vi "command_processor.vi"(8 "error in (no error)":errorcluster) -> (0 "error out":errorcluster)   [LabVIEW 2021]
uses:
  FGVs/FGVstates.ctl
  <vilib>/sound2/lvsound2.llb/Sampling Mode.ctl
  FGVs/AppStates.ctl
  <vilib>/sound2/lvsound2.llb/Sound Output Task ID.ctl
  <vilib>/sound2/lvsound2.llb/Sound File Position.ctl
  <vilib>/sound2/lvsound2.llb/Sound File Info (path).vi
  <vilib>/sound2/lvsound2.llb/Sound File Read Open.vi
  <vilib>/sound2/lvsound2.llb/Sound File Read (DBL).vi
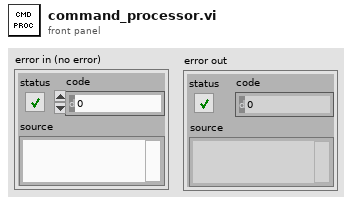
[diagram p1: front panel]
types:
  T1 = typedef "FGVstates.ctl" = enum16{"Init", "Set", "Get", "De-Init"}
  T2 = typedef "settings.ctl" = cluster{"scan_dir_path":path, "Number of Samples/Iteration":i32}
  T3 = typedef "data_exchange_fgv.ctl" = cluster{"queue states":refnum<queue>, "audio data":refnum<queue>, "error queue":refnum<queue>}
  T4 = typedef "AppStates.ctl" = enum16{"Init", "Scan Music Dir", "Idle", "Playback", "Enqueue samples", "Pause playback", "Stop playback", "Exit"}
  T5 = typedef "Sound Output Task ID.ctl" = u32
  T6 = typedef "ButtonRefs.ctl" = cluster{"Button_play":refnum<vi>, "Button_pause":refnum<vi>, "Button_stop":refnum<vi>, "Playback status":refnum<vi>, "Playback Timeline":refnum<vi>, "Right Channel":refnum<vi>, "Left Channel":refnum<vi>, "Skip Forward Button":refnum<vi>, "Skip Back Button":refnum<vi>, "Playlist":refnum<vi>}
  T7 = typedef "Sampling Mode.ctl" = i32
  T8 = typedef "Sound Data Format.ctl" = cluster{"sample rate (S/s)":dbl, "number of channels":i32, "bits per sample":i32}
  T9 = typedef "Sound File Refnum.ctl" = refnum<file>
  T10 = typedef "Sound File Position.ctl" = u16
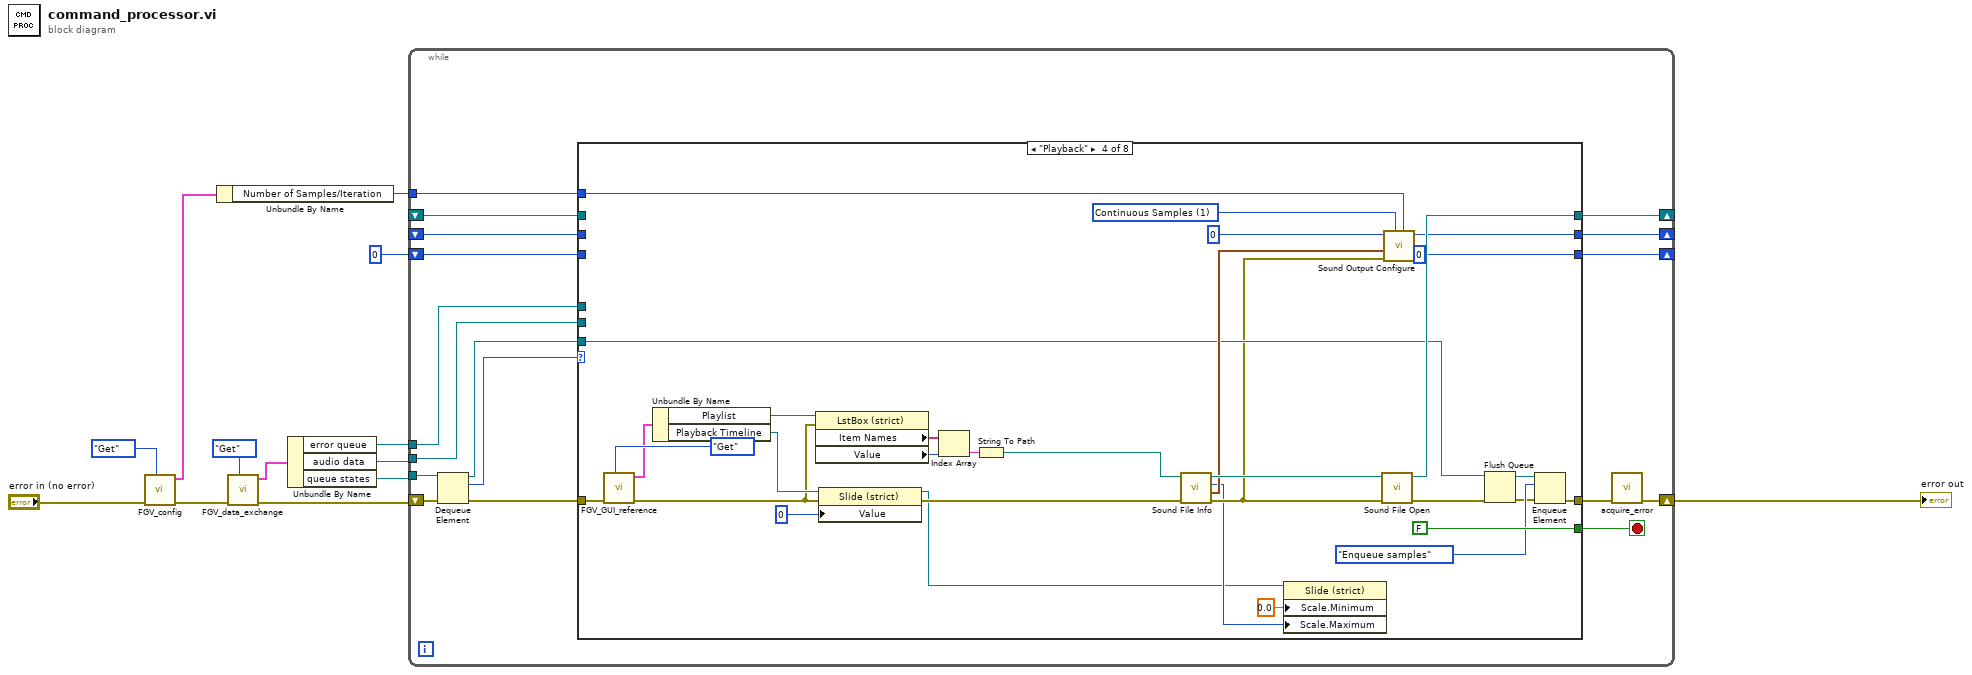
[diagram p0: block diagram]
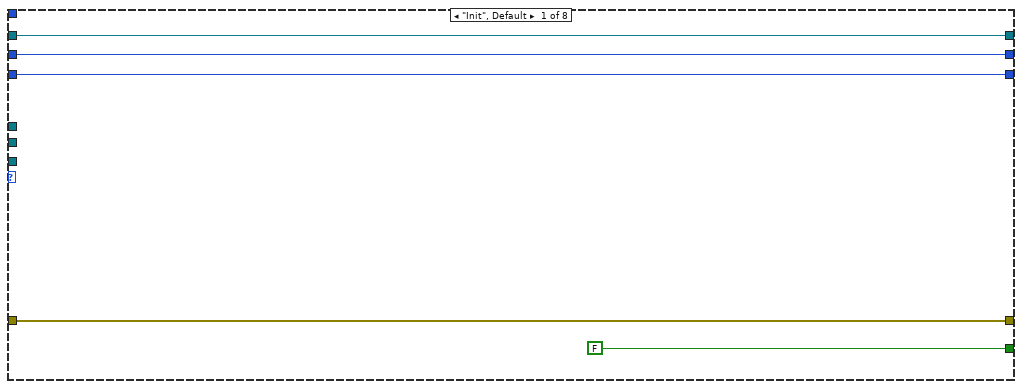
[diagram p2: hidden frame]
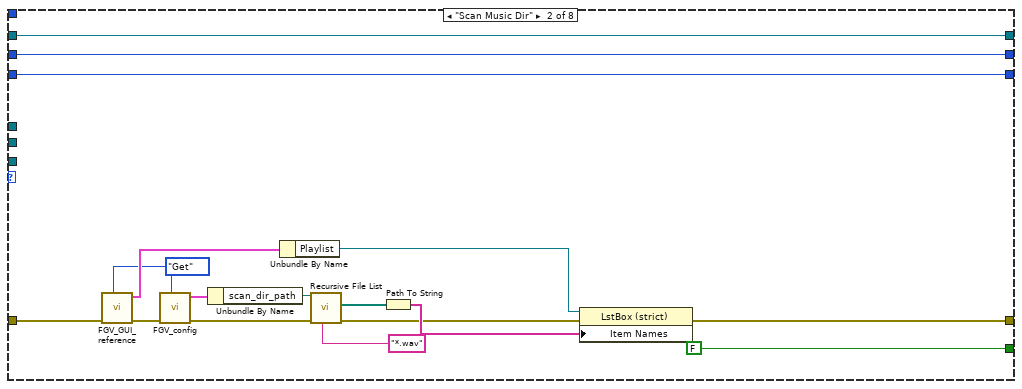
[diagram p3: hidden frame]
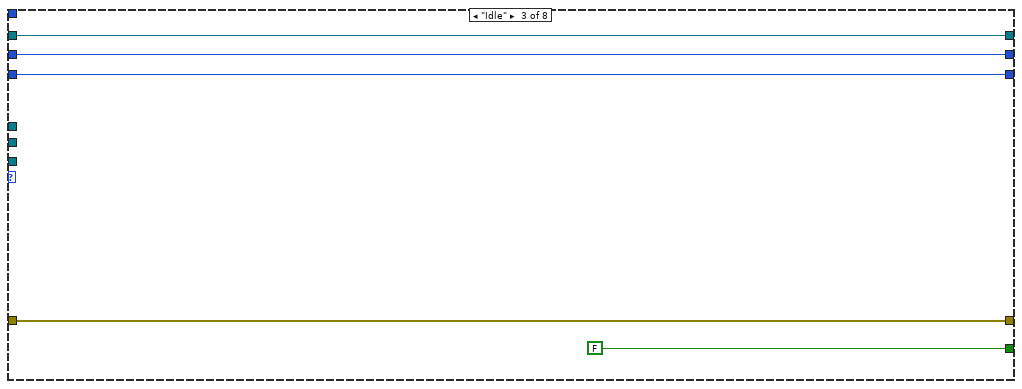
[diagram p4: hidden frame]
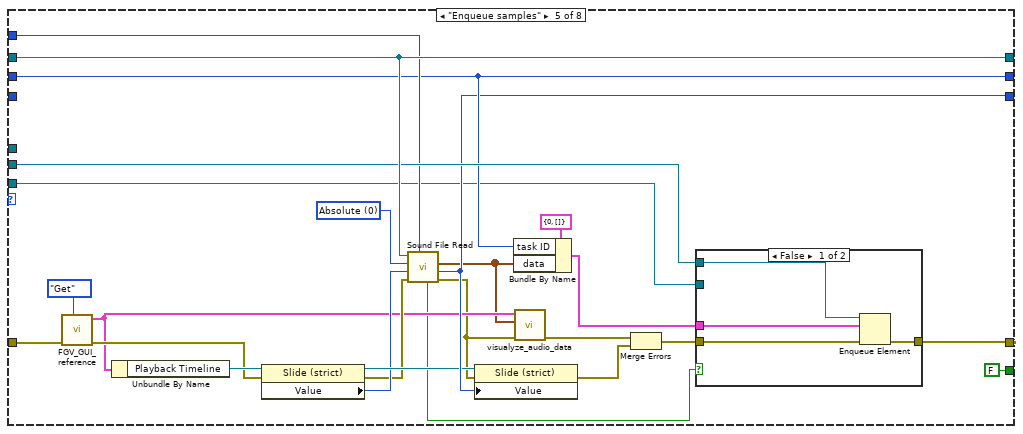
[diagram p5: hidden frame]
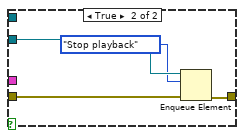
[diagram p6: hidden frame]
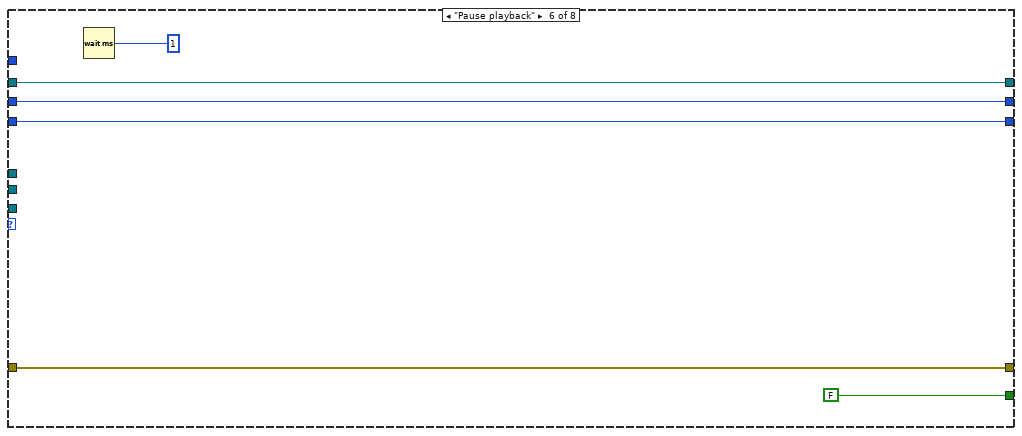
[diagram p7: hidden frame]
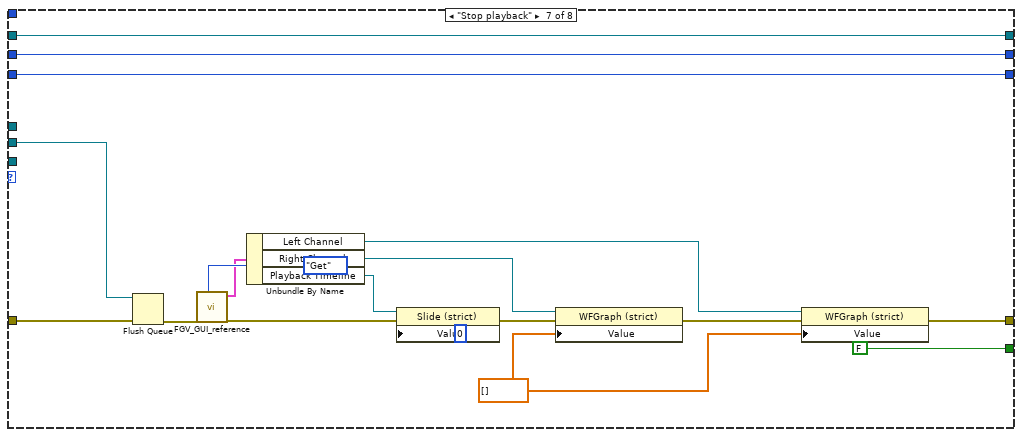
[diagram p8: hidden frame]
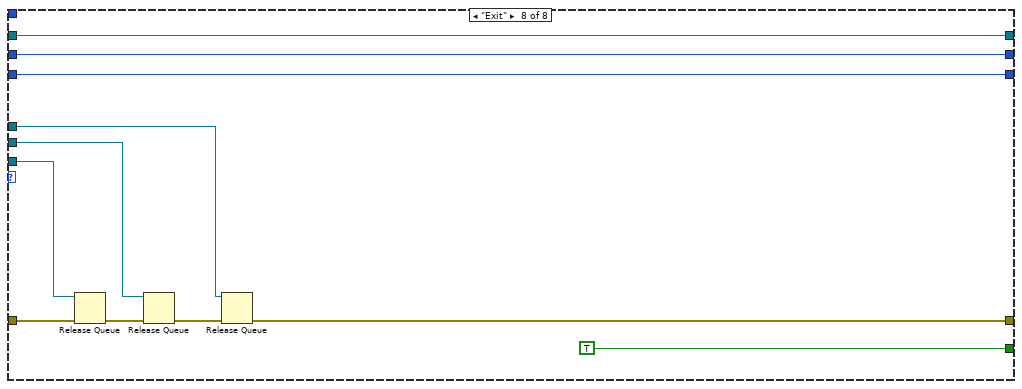
[diagram p9: hidden frame]
diagram:
  n1 = call "FGV_config.vi"("FGV states"=FGVstates."Get", "error in (no error)"="error in (no error)") -> ("error out"=w4:errorcluster, "Settings"=w2:T2)  [unwired: 8 in]
  n2 = Unbundle By Name(w2) -> ("Number of Samples/Iteration"=w1:i32)
  n3 = call "FGV_data_exchange.vi"("FGV states"=FGVstates."Get", "error in (no error)"=w4) -> ("error out"=w10:errorcluster, "main_cycle_queue"=w11:T3)  [unwired: 8 in]
  n4 = Unbundle By Name(w11) -> ("error queue"=w6:refnum<queue>, "audio data"=w8:refnum<queue>, "queue states"=w9:refnum<queue>)
  n5 = while {
    shift-right: [w15] -> w13
    shift-left: w10 -> [w30]
    tunnel: w9 -> [w26]
    shift-right: [w25] -> _
    shift-left: _ -> [w24]
    shift-right: [w23] -> _
    shift-left: _ -> [w22]
    tunnel: w1 -> [w20]
    tunnel: w8 -> [w19]
    shift-right: [w17] -> _
    shift-left: 0 ("position offset") -> [w18]
    tunnel: w6 -> [w14]
    stop <- w27 stop-if-true
    n6 = Dequeue Element(queue=w26, error in (no error)=w30) -> (queue out=w21:refnum<queue>, element=w29:T4, error out=w28:errorcluster)  [unwired: 1 in, 1 out]
    n7 = case shown="\"Playback\"" w29 {
      tunnel: w28 -> [w35 w50 w57 w88 w103 w122 w129 w152]
      tunnel: [w35 w36 w57 w74 w106 w122 w133 w146] -> w16
      tunnel: [FALSE FALSE FALSE FALSE FALSE FALSE FALSE TRUE] -> w27
      tunnel: [w32 w44 w54 w78 w112 w127 w145 w155] -> w25
      tunnel: w24 -> [w32 w44 w54 _ w112 w127 w145 w155]
      tunnel: [w33 w45 w55 w75 w108 w126 w144 w154] -> w23
      tunnel: w22 -> [w33 w45 w55 _ w108 w126 w144 w154]
      tunnel: w21 -> [_ _ _ w65 w89 _ _ w150]
      tunnel: w20 -> [_ _ _ w72 w110 _ _ _]
      tunnel: w19 -> [_ _ _ _ w111 _ w128 w149]
      tunnel: w18 -> [w31 w43 w53 _ _ w123 w143 w153]
      tunnel: [w31 w43 w53 0 ("position offset") w102 w123 w143 w153] -> w17
      tunnel: w14 -> [_ _ _ _ _ _ _ w147]
      frame "Init", Default {
      }
      frame "Scan Music Dir" {
        w41 = FGVstates."Get" ("FGV states")
        n8 = call "FGV_GUI_reference.vi"("FGV states"=w41, "error in (no error)"=w50) -> ("error out"=w42:errorcluster, "Button refs Out"=w49:T6)  [unwired: 8 in]
        n9 = call "FGV_config.vi"("FGV states"=w41, "error in (no error)"=w42) -> ("error out"=w40:errorcluster, "Settings"=w39:T2)  [unwired: 8 in]
        n10 = Unbundle By Name(w39) -> ("scan_dir_path"=w38:path)
        n11 = Unbundle By Name(w49) -> ("Playlist"=w46:refnum<vi>)
        n12 = call <vilib>:"Recursive File List.vi"("pattern"="*.wav", "error in (no error)"=w40, "Folder Path"=w38) -> ("error out"=w37:errorcluster, "All Files in Dir"=w48:path[])  [unwired: 4 in, 3 out]
        n13 = Path To String(path=w48) -> (string=w47:string[])
        n14 = property class="LstBox (strict)"(reference=w46, error in=w37, "Item Names"=w47) -> (error out=w36:errorcluster)  [unwired: 1 out]
      }
      frame "Idle" {
      }
      frame "Playback" {
        w77 = T7 1 items=["Finite Samples", "Continuous Samples"] ("sample mode")
        n15 = call "FGV_GUI_reference.vi"("FGV states"=FGVstates."Get", "error in (no error)"=w88) -> ("error out"=w64:errorcluster, "Button refs Out"=w86:T6)  [unwired: 8 in]
        n16 = Unbundle By Name(w86) -> ("Playlist"=w85:refnum<vi>, "Playback Timeline"=w69:refnum<vi>)
        n17 = property class="LstBox (strict)"(reference=w85, error in=w64) -> ("Item Names"=w82:string[], "Value"=w83:i32)  [unwired: 2 out]
        n18 = property class="Slide (strict)"(reference=w69, error in=w64, "Value"=0) -> (reference out=w58:refnum<vi>, error out=w63:errorcluster)
        n19 = Index Array(array=w82, index=w83) -> (element=w81:string)
        n20 = String To Path(string=w81) -> (path=w79:path)
        n21 = call-poly <vilib>:"Sound File Info.vi"("error in (no error)"=w63, "path"=w79) -> ("error out"=w62:errorcluster, "sound format"=w71:T8, "total number of samples/ch"=w59:u32, "path out"=w80:path)  [unwired: 6 in]
        n22 = property class="Slide (strict)"(reference=w58, "Scale.Minimum"=0.0 ("Scale.Range:Minimum"), "Scale.Maximum"=w59) -> ()  [unwired: 1 in, 2 out]
        n23 = call-poly <vilib>:"Sound File Open.vi"("error in (no error)"=w62, "path"=w80) -> ("error out"=w61:errorcluster, "sound file refnum"=w78:T9)  [unwired: 8 in]
        n24 = call <vilib>:"Sound Output Configure.vi"("number of samples/ch"=w72, "sample mode"=w77, "error in (no error)"=w62, "sound format"=w71, "device ID"=u32 0) -> ("task ID"=w75:T5)  [unwired: 5 in, 1 out]
        n25 = Flush Queue(queue=w65, error in (no error)=w61) -> (queue out=w66:refnum<queue>, error out=w67:errorcluster)  [unwired: 1 out]
        n26 = Enqueue Element(queue=w66, element=AppStates."Enqueue samples", error in (no error)=w67) -> (error out=w74:errorcluster)  [unwired: 1 in, 2 out]
      }
      frame "Enqueue samples" {
        w105 = T10 0 items=["Absolute"=0, "Relative"=2] ("position mode")
        n27 = call "FGV_GUI_reference.vi"("FGV states"=FGVstates."Get", "error in (no error)"=w103) -> ("error out"=w97:errorcluster, "Button refs Out"=w96:T6)  [unwired: 8 in]
        n28 = Unbundle By Name(w96) -> ("Playback Timeline"=w100:refnum<vi>)
        n29 = property class="Slide (strict)"(reference=w100, error in=w97) -> (reference out=w101:refnum<vi>, error out=w98:errorcluster, "Value"=w99:i32)
        n30 = call-poly <vilib>:"Sound File Read.vi"("number of samples/ch (-1: all)"=w110, "error in (no error)"=w98, "position offset"=w99, "position mode"=w105, "sound file refnum"=w112) -> ("error out"=w91:errorcluster, "offset"=w102:i32, "data"=w95:waveform(dbl)[], "end of file?"=w90:bool)  [unwired: 2 in, 1 out]
        n31 = property class="Slide (strict)"(reference=w101, error in=w91, "Value"=w102) -> (error out=w94:errorcluster)  [unwired: 1 out]
        n32 = Bundle By Name(cluster=cluster{"task ID":T5, "data":waveform(dbl)[]} {"task ID"=0, "data"=[]} ("element"), "task ID"=w108, "data"=w95) -> (w107:cluster{"task ID":T5, "data":waveform(dbl)[]})
        n33 = call "visualyze_audio_data.vi"("error in (no error)"=w91, "audio data"=w95, "Button refs In"=w96) -> ("error out"=w93:errorcluster)  [unwired: 8 in]
        n34 = Merge Errors(w93, w94) -> (w92:errorcluster)
        n35 = case shown="False" w90 {
          tunnel: w111 -> [w117 _]
          tunnel: w107 -> [w116 _]
          tunnel: [w115 w120] -> w106
          tunnel: w92 -> [w114 w118]
          tunnel: w89 -> [_ w121]
          frame False {
            n36 = Enqueue Element(queue=w117, element=w116, error in (no error)=w114) -> (error out=w115:errorcluster)  [unwired: 1 in, 2 out]
          }
          frame True {
            n37 = Enqueue Element(queue=w121, element=AppStates."Stop playback", error in (no error)=w118) -> (error out=w120:errorcluster)  [unwired: 1 in, 2 out]
          }
        }
      }
      frame "Pause playback" {
        n38 = Wait (ms)(milliseconds to wait=u32 1) -> ()  [unwired: 1 out]
      }
      frame "Stop playback" {
        w135 = dbl[] [] ("Value")
        n39 = Flush Queue(queue=w128, error in (no error)=w129) -> (error out=w130:errorcluster)  [unwired: 2 out]
        n40 = call "FGV_GUI_reference.vi"("FGV states"=FGVstates."Get", "error in (no error)"=w130) -> ("error out"=w137:errorcluster, "Button refs Out"=w141:T6)  [unwired: 8 in]
        n41 = Unbundle By Name(w141) -> ("Left Channel"=w131:refnum<vi>, "Right Channel"=w132:refnum<vi>, "Playback Timeline"=w140:refnum<vi>)
        n42 = property class="Slide (strict)"(reference=w140, error in=w137, "Value"=0) -> (error out=w134:errorcluster)  [unwired: 1 out]
        n43 = property class="WFGraph (strict)"(reference=w132, error in=w134, "Value"=w135) -> (error out=w136:errorcluster)  [unwired: 1 out]
        n44 = property class="WFGraph (strict)"(reference=w131, error in=w136, "Value"=w135) -> (error out=w133:errorcluster)  [unwired: 1 out]
      }
      frame "Exit" {
        n45 = Release Queue(queue=w150, error in (no error)=w152) -> (error out=w151:errorcluster)  [unwired: 1 in, 2 out]
        n46 = Release Queue(queue=w149, error in (no error)=w151) -> (error out=w148:errorcluster)  [unwired: 1 in, 2 out]
        n47 = Release Queue(queue=w147, error in (no error)=w148) -> (error out=w146:errorcluster)  [unwired: 1 in, 2 out]
      }
    }
    n48 = call "acquire_error.vi"("error in (no error)"=w16) -> ("error out"=w15:errorcluster)  [unwired: 10 in]
  }
  "error out" <- w13
